vi "GETPCID.vi"() -> ()   [LabVIEW 2013]
panel:
  in  "Btn_GetID":bool
  out "ID":string
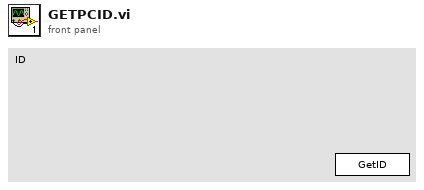
[diagram p1: front panel]
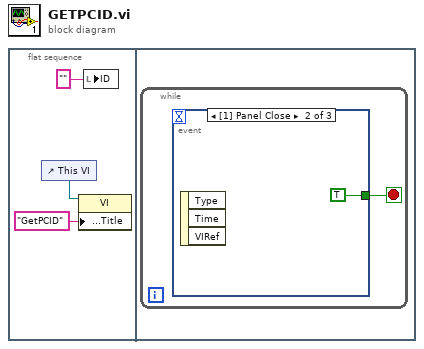
[diagram p0: block diagram]
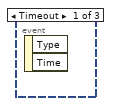
[diagram p2: hidden frame]
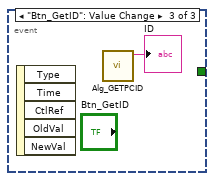
[diagram p3: hidden frame]
diagram:
  n1 = flat-sequence {
    frame #0 {
      n2 = control-ref of="This VI"() -> (w2:refnum<vi>)
      n3 = property class="VI"(reference=w2, "Front Panel.Title"="GetPCID" ("Front Panel Window:Title")) -> ()  [unwired: 1 in, 2 out]
      n4 = local write "ID"("" ("ID")) -> ()
    }
    frame #1 {
      n5 = while {
        stop <- w4 stop-if-true
        n6 = event shown="[1] Panel Close" {
          selector: _ -> [_ _ _]
          dyn-events: _ -> [_ _ _]
          timeout: _ -> [_ _ _]
          tunnel: [_ TRUE _] -> w4
          event Timeout {
            n7 = event-data() -> ()  [unwired: 1 in, 2 out]
          }
          event Panel Close {
            n8 = event-data() -> ()  [unwired: 1 in, 3 out]
          }
          event "Btn_GetID": Value Change {
            n9 = event-data() -> ()  [unwired: 1 in, 5 out]
            n10 = call "Alg_GETPCID.vi"() -> ("ID"=→"ID":string)  [unwired: 11 in]
          }
        }
      }
    }
  }
